vi "ReloadINIFiles.vi"(8 "error in (no error)":errorcluster, 11 "ModuleID":i32) -> (0 "error out":errorcluster)   [LabVIEW 2014, in "MyPlugins.lvlib" / "MyPluginsBase.lvclass"]
doc: "This VI broadcast a message from the plugin to the module in order for the module to reload the INI files to show any new PluginTypes associated with the any new INI file created."
uses:
  MyPluginsBase.lvclass
  MyPluggableModule/PublicAPI/Requests/clEventType.ctl
  <vilib>/Utility/error.llb/Error Cluster From Error Code.vi
  <vilib>/ErrorRing/Error Ring.xnode
  MyPluggableModule/MyPluggableModule.lvlib
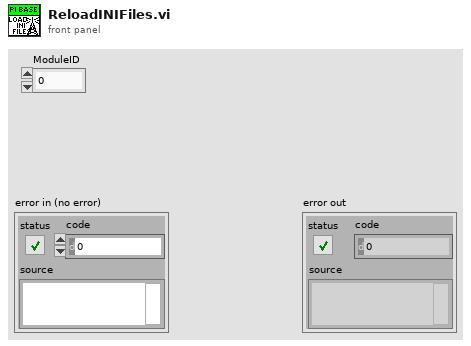
[diagram p1: front panel]
types:
  T1 = typedef "MyPluggableModule.lvlib/clBroadcastEvents.ctl" = cluster{"DidInit":refnum<user-event>, "StatusUpdate":refnum<user-event>, "ErrorReport":refnum<user-event>, "DidStop":refnum<user-event>, "PathToINI":refnum<user-event>, "ReloadINIFiles":refnum<user-event>}
  T2 = typedef "MyPluggableModule.lvlib/clEventType.ctl" = cluster{"ModuleID":i32, "Data":variant}
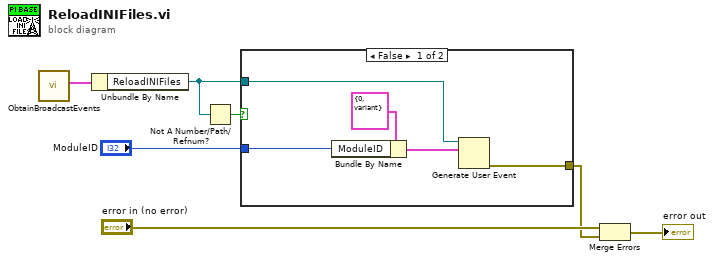
[diagram p0: block diagram]
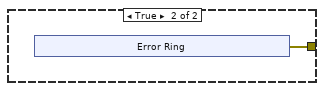
[diagram p2: hidden frame]
diagram:
  n1 = call "ObtainBroadcastEvents.vi"() -> ("clBroadcastEvents"=w7:T1)  [unwired: 10 in, 1 out]
  n2 = Unbundle By Name(w7) -> ("ReloadINIFiles"=w2:refnum<user-event>)
  n3 = Not A Number/Path/Refnum?(number/path/refnum=w2) -> (NaN/Path/Refnum?=w3:bool)
  n4 = case shown="False" w3 {
    tunnel: "ModuleID" -> [w11 _]
    tunnel: w2 -> [w9 _]
    tunnel: [w8 w13] -> w1
    frame False {
      n5 = Bundle By Name(cluster=T2 {"ModuleID"=0, "Data"=variant} ("clEventType"), "ModuleID"=w11) -> (w10:T2)
      n6 = Generate User Event(user event=w9, event data cluster=w10) -> (error out=w8:errorcluster)  [unwired: 2 in, 1 out]
    }
    frame True {
      n7 = xnode "Error Ring"() -> ("error out"=w13:errorcluster)
    }
  }
  n8 = Merge Errors("error in (no error)", w1) -> (→"error out":errorcluster)
